vi "Enable or Gray Out.vi"(1 "Boolean":bool) -> (0 "Disabled":T1(ring))   [LabVIEW 2020]
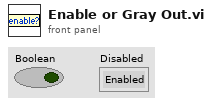
[diagram p1: front panel]
types:
  T1 = enum8{"Enabled", "Disabled", "Disabled and Grayed Out"}
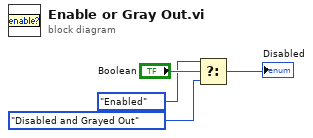
[diagram p0: block diagram]
diagram:
  n1 = Select(t=T1."Enabled" ("Disabled"), s="Boolean", f=T1."Disabled and Grayed Out" ("Disabled")) -> (s? t:f=→"Disabled":T1)
